vi "Black Start.vi"(8 "error in (no error)":errorcluster, 10 "Sequence":string, 11 "SCADA in":refnum<class "SCADA.lvclass">) -> (0 "error out":errorcluster, 3 "SCADA out":refnum<class "SCADA.lvclass">)   [LabVIEW 2015, in "SCADA Core.lvlib" / "SCADA.lvclass"]
uses:
  SCADA.lvclass
  SCADA.lvclass/SCADA.ctl
  IED Actor/IED/Controls/Generation Mode.ctl
  Controls/Grid Mode.ctl
  SCADA Messages/Log Msg/Log Msg.lvclass
  SCADA Messages/Measurement Visualization Msg/Measurement Visualization Msg.lvclass
  <vilib>/ActorFramework/Actor/Actor.lvclass/Actor.ctl
  <vilib>/ActorFramework/Message Enqueuer/Message Enqueuer.lvclass/Message Enqueuer.ctl
  IED Actor/IED Messages/Set Generation Mode Msg/Set Generation Mode Msg.lvclass/Set Generation Mode Msg.ctl
  IED Actor/IED/Controls/Device Deactivate Mode Select.ctl
  IED Actor/IED Messages/Device Deactivate Msg/Device Deactivate Msg.lvclass/Device Deactivate Msg.ctl
  SCADA Messages/Set Number of Activations Msg/Set Number of Activations Msg.lvclass/Set Number of Activations Msg.ctl
  IED Actor/IED/Controls/Device Activate Mode Select.ctl
  SCADA Action Messages/Device Activate Msg/Device Activate Msg.lvclass/Device Activate Msg.ctl
  SCADA Abstract Messages/Black Start Status Msg/Black Start Status.ctl
  <vilib>/Utility/error.llb/DialogType.ctl
  SCADA Messages/Return Black Start Status Msg/Return Black Start Status Msg.lvclass/Return Black Start Status Msg.ctl
  <vilib>/ActorFramework/Message Enqueuer/Init from Existing Queue.vi
  <vilib>/ActorFramework/Message Enqueuer/Enqueue.vi
  <vilib>/ActorFramework/Message Priority Queue/Priority Enqueue.vi
  <vilib>/ActorFramework/Message Enqueuer/Message Enqueuer.lvclass
  IED Actor/IED Messages/Set Generation Mode Msg/Set Generation Mode Msg.lvclass
  IED Actor/IED Messages/Device Deactivate Msg/Device Deactivate Msg.lvclass
  SCADA Messages/Set Number of Activations Msg/Set Number of Activations Msg.lvclass
  SCADA Action Messages/Device Activate Msg/Device Activate Msg.lvclass
  SCADA Messages/Return Black Start Status Msg/Return Black Start Status Msg.lvclass
  <vilib>/ActorFramework/Actor/Actor.lvclass
  IED Actor/IED/IED.lvclass
  SCADA Abstract Messages/Black Start Status Msg/Black Start Status Msg.lvclass
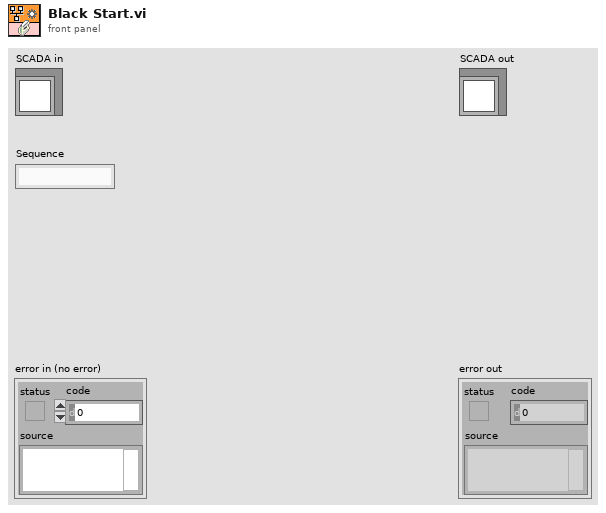
[diagram p1: front panel]
types:
  T1 = typedef "SCADA Core.lvlib/SCADA.lvclass/Grid Mode.ctl" = enum16{"Off", "Grid Connected", "Islanded", "Synchronizing"}
  T2 = typedef "IED Actor.lvlib/IED.lvclass/Generation Mode.ctl" = enum16{"P/Q", "V/f"}
  T3 = typedef "IED Actor.lvlib/IED.lvclass/Device Activate Mode Select.ctl" = enum16{"Activate", "Blackstart", "Individual"}
  T4 = typedef "IED Actor.lvlib/IED.lvclass/Device Deactivate Mode Select.ctl" = enum16{"Deactivate", "Shutdown", "Island"}
  T5 = typedef "SCADA Core.lvlib/Black Start Status Msg.lvclass/Black Start Status.ctl" = enum16{"Success", "Failure"}
  T6 = typedef "DialogType.ctl" = u16
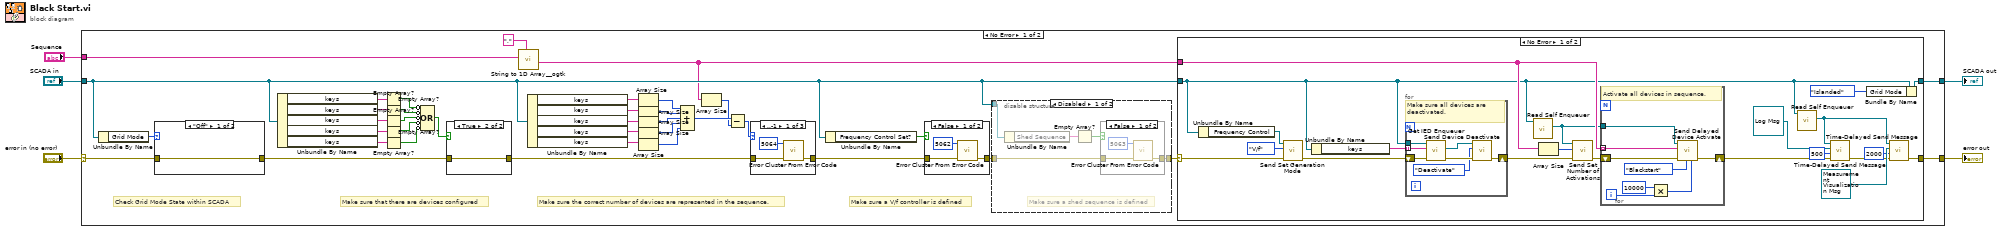
[diagram p0: block diagram]
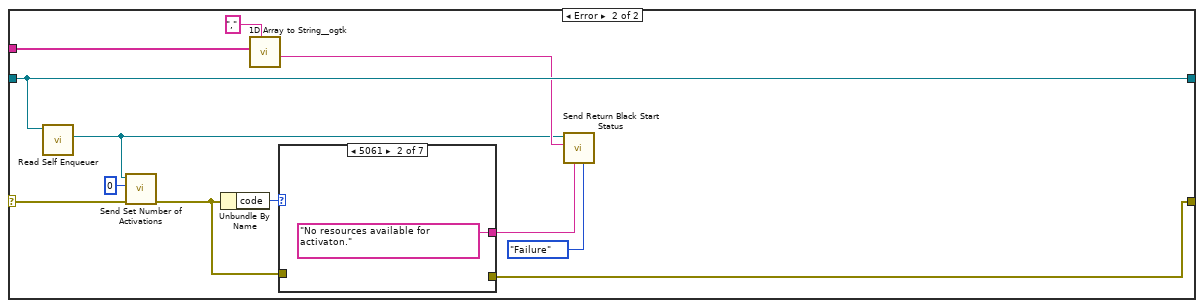
[diagram p2: hidden frame]
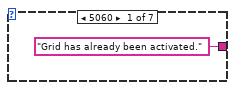
[diagram p3: hidden frame]
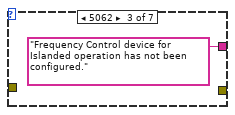
[diagram p4: hidden frame]
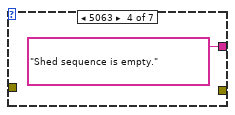
[diagram p5: hidden frame]
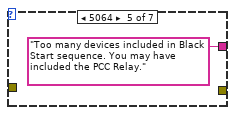
[diagram p6: hidden frame]
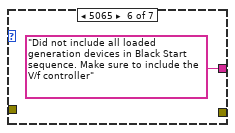
[diagram p7: hidden frame]
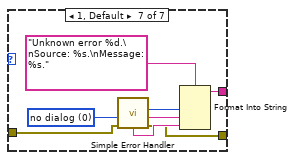
[diagram p8: hidden frame]
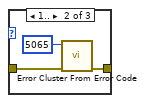
[diagram p11: hidden frame]
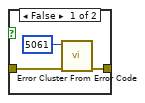
[diagram p14: hidden frame]
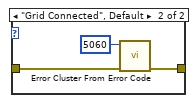
[diagram p15: hidden frame]
diagram:
  n1 = case shown="No Error" "error in (no error)" {
    selector: "error in (no error)" -> [w42 w136]
    tunnel: [w37 w136] -> w4
    tunnel: [w38 w135] -> w2
    tunnel: "SCADA in" -> [w18 w135]
    tunnel: "Sequence" -> [w17 _]
    frame No Error {
      # "Make sure a V/f controller is defined"
      # "Make sure the correct number of devices are represented in the sequence."
      # "Make sure that there are devices configured"
      # "Check Grid Mode State within SCADA"
      n2 = Unbundle By Name(w18) -> ("Grid Mode"=w43:T1)
      n3 = case shown="\"Off\"" w43 {
        tunnel: w42 -> [w131 w134]
        tunnel: [w131 w132] -> w41
        frame "Off" {
        }
        frame "Grid Connected", Default {
          n4 = call <vilib>:"Error Cluster From Error Code.vi"("error in (no error)"=w134, "error code (0)"=5060) -> ("error out"=w132:errorcluster)  [unwired: 7 in]
        }
      }
      n5 = Unbundle By Name(w18) -> ("keys"=w35:string[], "keys"=w32:string[], "keys"=w33:string[], "keys"=w34:string[], "keys"=w9:string[])
      n6 = Empty Array?(array=w35) -> (empty?=w31:bool)
      n7 = Empty Array?(array=w32) -> (empty?=w30:bool)
      n8 = Empty Array?(array=w33) -> (empty?=w29:bool)
      n9 = Empty Array?(array=w34) -> (empty?=w28:bool)
      n10 = Empty Array?(array=w9) -> (empty?=w8:bool)
      n11 = Compound Arithmetic op=OR(invert w31, invert w30, invert w29, invert w28, invert w8) -> (w40:bool)
      n12 = case shown="True" w40 {
        tunnel: w41 -> [w129 w130]
        tunnel: [w127 w130] -> w12
        frame False {
          n13 = call <vilib>:"Error Cluster From Error Code.vi"("error in (no error)"=w129, "error code (0)"=5061) -> ("error out"=w127:errorcluster)  [unwired: 7 in]
        }
        frame True {
        }
      }
      n14 = call <userlib>:"String to 1D Array__ogtk.vi"("delimiter (Tab)"=",", "string"=w17) -> ("Array of Strings"=w10:string[])  [unwired: 9 in]
      n15 = Unbundle By Name(w18) -> ("keys"=w26:string[], "keys"=w25:string[], "keys"=w24:string[], "keys"=w23:string[], "keys"=w7:string[])
      n16 = Array Size(array=w26) -> (size(s)=w22:i32)
      n17 = Array Size(array=w25) -> (size(s)=w21:i32)
      n18 = Array Size(array=w24) -> (size(s)=w20:i32)
      n19 = Array Size(array=w23) -> (size(s)=w19:i32)
      n20 = Array Size(array=w7) -> (size(s)=w6:i32)
      n21 = Compound Arithmetic op=ADD(w22, w21, w20, w19, w6) -> (w15:i32)
      n22 = Array Size(array=w10) -> (size(s)=w14:i32)
      n23 = Subtract(x=w15, y=w14) -> (x-y=w13:i32)
      n24 = case shown="..-1" w13 {
        tunnel: w12 -> [w118 w121 w122]
        tunnel: [w116 w119 w122] -> w11
        frame ..-1 {
          n25 = call <vilib>:"Error Cluster From Error Code.vi"("error in (no error)"=w118, "error code (0)"=5064) -> ("error out"=w116:errorcluster)  [unwired: 7 in]
        }
        frame 1.. {
          n26 = call <vilib>:"Error Cluster From Error Code.vi"("error in (no error)"=w121, "error code (0)"=5065) -> ("error out"=w119:errorcluster)  [unwired: 7 in]
        }
        frame 0 {
        }
      }
      n27 = Unbundle By Name(w18) -> ("Frequency Control Set?"=w39:bool)
      n28 = case shown="False" w39 {
        tunnel: w11 -> [w125 w126]
        tunnel: [w123 w126] -> w36
        frame False {
          n29 = call <vilib>:"Error Cluster From Error Code.vi"("error in (no error)"=w125, "error code (0)"=5062) -> ("error out"=w123:errorcluster)  [unwired: 7 in]
        }
        frame True {
        }
      }
      n30 = disable-structure shown="Disabled" {
        disable-tunnel: w36 -> [w110 w115]
        disable-tunnel: [w107 w115] -> w27
        disable-tunnel: w18 -> [w106 _]
        frame Disabled {
          # "Make sure a shed sequence is defined"
          n31 = Unbundle By Name(w106) -> ("Shed Sequence"=w108:string[])
          n32 = Empty Array?(array=w108) -> (empty?=w109:bool)
          n33 = case shown="False" w109 {
            tunnel: w110 -> [w113 w114]
            tunnel: [w111 w114] -> w107
            frame False {
              n34 = call <vilib>:"Error Cluster From Error Code.vi"("error in (no error)"=w113, "error code (0)"=5063) -> ("error out"=w111:errorcluster)  [unwired: 7 in]
            }
            frame True {
            }
          }
        }
        frame Enabled {
          # "We aren't implementing Shed yet."
        }
      }
      n35 = case shown="No Error" w27 {
        selector: w27 -> [w57 w86]
        tunnel: w18 -> [w44 w90]
        tunnel: [w54 w90] -> w38
        tunnel: [w45 w80] -> w37
        tunnel: w10 -> [w61 w89]
        frame No Error {
          n36 = Unbundle By Name(w44) -> ("Frequency Control"=w58:refnum<class "Message Enqueuer.lvclass">)
          n37 = call "Send Set Generation Mode.vi"("error in (no error)"=w57, "Mode"=Generation_Mode."V/f", "Message Enqueuer"=w58) -> ("error out"=w56:errorcluster)  [unwired: 7 in, 1 out]
          n38 = Unbundle By Name(w44) -> ("keys"=w64:string[])
          n39 = for {
            tunnel: w44 -> [w79]
            tunnel: w64 -> [w78] mode=indexing
            shift-right: [w74] -> w63
            shift-left: w56 -> [w77]
            # "Make sure all devices are deactivated."
            n40 = call "Get IED Enqueuer.vi"("error in (no error)"=w77, "IED Name"=w78, "SCADA in"=w79) -> ("error out"=w76:errorcluster, "IED Enqueuer"=w75:refnum<class "Message Enqueuer.lvclass">)  [unwired: 6 in, 1 out]
            n41 = call "Send Device Deactivate.vi"("error in (no error)"=w76, "Activate Mode"=Device_Deactivate_Mode_Select."Deactivate", "Message Enqueuer"=w75) -> ("error out"=w74:errorcluster)  [unwired: 7 in, 1 out]
          }
          n42 = call <vilib>:"Read Self Enqueuer.vi"("Actor"=w44) -> ("Self Enqueuer"=w59:refnum<class "Message Enqueuer.lvclass">)  [unwired: 10 in]
          n43 = Array Size(array=w61) -> (size(s)=w60:i32)
          n44 = call "Send Set Number of Activations.vi"("error in (no error)"=w63, "Number of Activations"=w60, "Message Enqueuer"=w59) -> ("error out"=w62:errorcluster)  [unwired: 7 in, 1 out]
          n45 = for {
            tunnel: w61 -> [w71] mode=indexing
            shift-right: [w69] -> w46
            shift-left: w62 -> [w70]
            tunnel: w59 -> [w72]
            i -> [w67]
            # "Activate all devices in sequence."
            n46 = Multiply(x=10000, y=w67) -> (x*y=w65:i32)
            n47 = call "Send Delayed Device Activate.vi"("Milliseconds To Wait"=w65, "Activate Mode"=Device_Activate_Mode_Select."Blackstart", "error in (no error)"=w70, "IED Name"=w71, "Message Enqueuer"=w72) -> ("error out"=w69:errorcluster)  [unwired: 6 in]
          }
          n48 = call <vilib>:"Read Self Enqueuer.vi"("Actor"=w44) -> ("Self Enqueuer"=w51:refnum<class "Message Enqueuer.lvclass">)  [unwired: 10 in]
          n49 = call <vilib>:"Time-Delayed Send Message.vi"("error in (no error)"=w46, "Milliseconds To Wait"=500, "Message"=refnum<class "Log Msg.lvclass"> refnum ("SCADA Core.lvlib:Log Msg.lvclass"), "Message Enqueuer"=w51) -> ("error out"=w50:errorcluster)  [unwired: 6 in, 1 out]
          n50 = Bundle By Name(cluster=w44, "Grid Mode"=Grid_Mode."Islanded") -> (w54:refnum<class "SCADA.lvclass">)
          n51 = call <vilib>:"Time-Delayed Send Message.vi"("error in (no error)"=w50, "Milliseconds To Wait"=2000, "Message"=refnum<class "Measurement Visualization Msg.lvclass"> refnum ("SCADA Core.lvlib:Measurement Visualization Msg.lvclass"), "Message Enqueuer"=w51) -> ("error out"=w45:errorcluster)  [unwired: 6 in, 1 out]
        }
        frame Error {
          n52 = call <vilib>:"Read Self Enqueuer.vi"("Actor"=w90) -> ("Self Enqueuer"=w84:refnum<class "Message Enqueuer.lvclass">)  [unwired: 10 in]
          n53 = call "Send Set Number of Activations.vi"("error in (no error)"=w86, "Number of Activations"=0, "Message Enqueuer"=w84) -> ("error out"=w85:errorcluster)  [unwired: 7 in, 1 out]
          n54 = Unbundle By Name(w85) -> ("code"=w91:i32)
          n55 = call <userlib>:"1D Array to String__ogtk.vi"("delimiter (Tab)"=",", "Array of Strings"=w89) -> ("delimited string"=w87:string)  [unwired: 9 in]
          n56 = case shown="5061" w91 {
            tunnel: w85 -> [_ _ _ _ _ _ w100]
            tunnel: ["Grid has already been activated." "No resources available for activaton." "Frequency Control device for Islanded operation has not been configured." "Shed sequence is empty." "Too many devices included in Black Start sequence. You may have included the PCC Relay." "Did not include all loaded generation devices in Black Start sequence. Make sure to include the V/f controller" w99] -> w81
            tunnel: [_ _ _ _ _ _ w98] -> w80
            frame 5060 {
            }
            frame 5061 {
            }
            frame 5062 {
            }
            frame 5063 {
            }
            frame 5064 {
            }
            frame 5065 {
            }
            frame 1, Default {
              w101 = T6 0 items=["no dialog", "OK message", "continue or stop message", "OK message + warnings", "continue/stop + warnings"] ("type of dialog (OK msg:1)")
              n57 = call <vilib>:"Simple Error Handler.vi"("type of dialog (OK msg:1)"=w101, "error in (no error)"=w100) -> ("code out"=w103:i32, "source out"=w104:string, "error out"=w98:errorcluster, "message"=w105:string)  [unwired: 3 in, 1 out]
              n58 = Format Into String(format string="Unknown error %d.\nSource: %s.\nMessage: %s." ("Error String"), w103, w104, w105) -> (resulting string=w99:string)  [unwired: 2 in, 1 out]
            }
          }
          n59 = call "Send Return Black Start Status.vi"("Status"=Black_Start_Status."Failure", "error"=w81, "IED Name"=w87, "Message Enqueuer"=w84) -> ()  [unwired: 6 in, 2 out]
        }
      }
    }
    frame Error {
    }
  }
  "error out" <- w4
  "SCADA out" <- w2
